vi "Download-Data.vi"() -> ()   [LabVIEW 2014]
doc: "This example performs a serial port write and a serial port read. The parameters set for the serial port must match the parameters of the connected instrument or device. The VISA Configure Serial Port VI sets the configuration parameters. The front panel displays the controls used to configure the basic parameters, such as baud rate, data bits, and parity. The VI passes the VISA resource name to other VIs that perform operations on that VISA resource. The VISA Write function sends a command to the serial device and the VISA Read function returns data based on the command. The VISA Close function then closes the reference to the serial device. It is important to close the reference; otherwise, further communication through that port might not be possible."
uses:
  Program Files (x86)/National Instruments/LabVIEW 2014/examples/Instrument IO/Serial/support/Serial - Settings.ctl
  <vilib>/Instr/_visa.llb/VISA Configure Serial Port (Instr).vi
  <vilib>/regexp/Match Regular Expression.xnode
panel:
  out "Humidity":dbl[](graph)
  out "Temperature":dbl[](graph)
  out "Downloading data":i32(slide) scale=0.0..254.0
  in  "VISA resource name":refnum<visa-resource-name>="COM3"
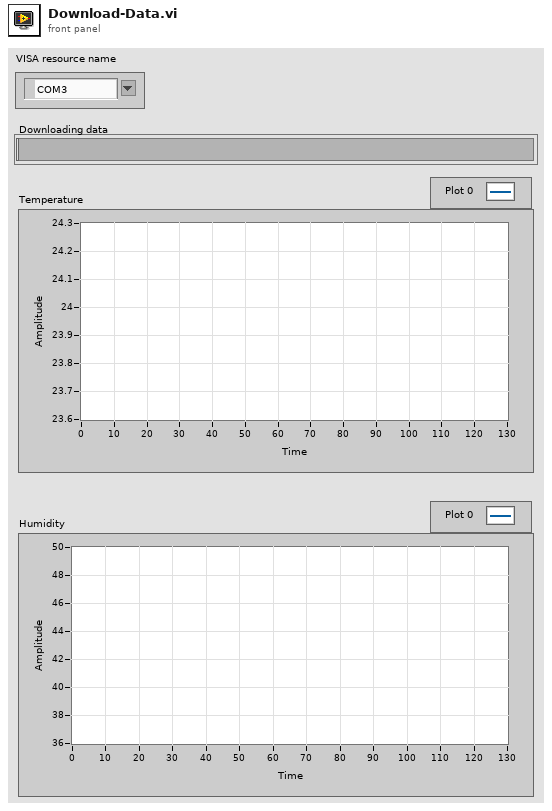
[diagram p1: front panel]
types:
  T1 = typedef "Serial - Settings.ctl" = cluster{"baud rate":u32, "data bits":u16, "parity":enum16{"None", "Odd", "Even", "Mark", "Space"}, "stop bits":u16, "flow control":u16}
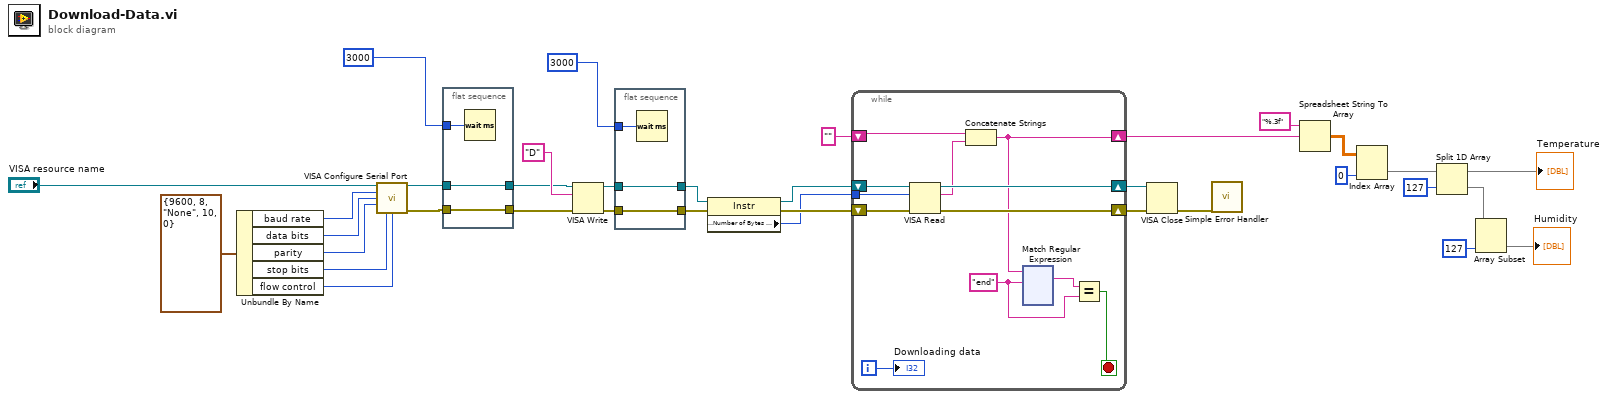
[diagram p0: block diagram]
diagram:
  n1 = Unbundle By Name(T1 {"baud rate"=9600, "data bits"=8, "parity"=enum."None", "stop bits"=10, "flow control"=0} ("Serial Settings")) -> ("baud rate"=w22:u32, "data bits"=w21:u16, "parity"=w20:enum16{"None", "Odd", "Even", "Mark", "Space"}, "stop bits"=w19:u16, "flow control"=w18:u16)
  n2 = call-poly "VISA Configure Serial Port"("VISA resource name"="VISA resource name", "baud rate (9600)"=w22, "data bits (8)"=w21, "parity (0:none)"=w20, "stop bits (10: 1 bit)"=w19, "flow control (0:none)"=w18) -> ("VISA resource name out"=w17:refnum<visa-resource-name>, "error out"=w14:errorcluster)  [unwired: 3 in, 5 out]
  n3 = flat-sequence {
    tunnel: w14 -> [w37]
    tunnel: [w37] -> w15
    tunnel: w17 -> [w36]
    tunnel: [w36] -> w16
    tunnel: u32 3000 ("delay before read (ms)") -> [w38]
    frame #0 {
      n4 = Wait (ms)(milliseconds to wait=w38) -> ()  [unwired: 1 out]
    }
  }
  n5 = VISA Write(VISA resource name=w16, write buffer="D" ("Command"), error in (no error)=w15) -> (VISA resource name out=w29:refnum<visa-resource-name>, error out=w31:errorcluster)  [unwired: 1 out]
  n6 = flat-sequence {
    tunnel: w31 -> [w40]
    tunnel: [w40] -> w30
    tunnel: w29 -> [w39]
    tunnel: [w39] -> w28
    tunnel: u32 3000 ("delay before read (ms)") -> [w41]
    frame #0 {
      n7 = Wait (ms)(milliseconds to wait=w41) -> ()  [unwired: 1 out]
    }
  }
  n8 = property class="Instr"(reference=w28, error in=w30) -> (reference out=w26:refnum<visa-resource-name>, error out=w25:errorcluster, "Serial Settings:Number of Bytes at Serial Port"=w24:u32)
  n9 = while {
    tunnel: w24 -> [w49]
    shift-right: [w52] -> w33
    shift-left: w26 -> [w51]
    shift-right: [w53] -> w34
    shift-left: w25 -> [w50]
    shift-right: [w46] -> w8
    shift-left: "" -> [w48]
    i -> [w42]
    stop <- w43 stop-if-true
    w44 = "end" ("regular expression")
    n10 = VISA Read(VISA resource name=w51, byte count=w49, error in (no error)=w50) -> (VISA resource name out=w52:refnum<visa-resource-name>, read buffer=w47:string, error out=w53:errorcluster)  [unwired: 1 out]
    n11 = Concatenate Strings(w48, w47) -> (w46:string)
    n12 = xnode "Match Regular Expression"("input string"=w46, "regular expression"=w44) -> ("whole match"=w45:string)  [unwired: 4 in, 4 out]
    n13 = Equal?(x=w45, y=w44) -> (x = y?=w43:bool)
    "Downloading data" <- w42
  }
  n14 = VISA Close(VISA resource name=w33, error in (no error)=w34) -> (error out=w32:errorcluster)
  n15 = call <vilib>:"Simple Error Handler.vi"("error in (no error)"=w32) -> ()  [unwired: 1 in, 8 out]
  n16 = Spreadsheet String To Array(format string="%.3f", spreadsheet string=w8) -> (array=w10:dbl[][])  [unwired: 2 in]
  n17 = Index Array(array=w10, index (col)=0 ("disabled index (col)")) -> (element=w4:dbl[])  [unwired: 1 in]
  n18 = Split 1D Array(array=w4, index=127) -> (first subarray=→"Temperature":dbl[], second subarray=w6:dbl[])
  n19 = Array Subset(array=w6, length=127) -> (→"Humidity":dbl[])  [unwired: 1 in]
